vi "SyncedRecording.vi"() -> ()   [LabVIEW 2017]
doc: "I. Description:\nThis example demonstrates how to continuously acquire and generate data at the same time, synchronized with one another.\n\nII. Instructions for Running:\n1. Select the physical channel to correspond to where your signal is input on the DAQ device. Also, select the corresponding channel for where your signal is being generated.\n2. Enter the minimum and maximum voltage ranges.\nNote: For better accuracy try to match the input range to the expected voltage level of the measured signal.\n3. Set the sample rate of the acquisition.\nNote: The rate should be at least twice as fast as the maximum frequency component of the signal being acquired. \n6. Select the Rate for the generation\n7. Select what type of signal to generate and the amplitude.\nNote: This example requires two DMA channels to run. If your hardware does not support two DMA channels, you need to set the Data Transfer Mechanism property for the Analog Output Task to use \"Interrupts\". The Data Transfer Mechanism property is located in the DAQmx Channel Property hierarchy at:\n\nDAQmx Channel Property Node>>Analog Output>>General Properties>>Advanced>>Data Transfer and Memory>>Data Transfer Mechanism\n\nRefer to your device documentation to determine how many DMA channels are supported for your hardware.\n\nIII. Block Diagram Steps:\n1. Create an analog input voltage channel. Also, create an analog output voltage channel.\n2. Set the rate for the sample clock. Additionally, define the sample mode to be continuous. Also, set the sample clock rate for the signal generation.\n2a. Call the Get Terminal Name with Device Prefix VI. This will take a Task and a terminal and create a properly formatted device + terminal name to use as the source of the Trigger.\n3. Define the parameters for a Digital Edge Start Trigger. Set the Analog output to trigger off the AI Start Trigger. This is an internal trigger signal.\n4. Use the Basic Function Generator VI to create the signal to be generated.\n5. Call the Start VI to arm the two functions. Make sure the analog output is armed before the analog input. This will ensure both will start at the same time.\n6. Read the waveform data in a loop until the user hits the stop button or an error occurs. The Is Task Done? VI is used to check for errors in the Analog Output Task.\n7. Call the Clear VI to Clear the Task\n8. Use the popup dialog box to display an error if any.\n\nIV. I/O Connections Overview:\nMake sure your signal input/output terminals match the Physical Channel I/O controls."
uses:
  <vilib>/measure/NI_MABase.lvlib
panel:
  in  "Analog Input Sample Clock Source":tag="/Dev1/ao/SampleClock"
  out "Actual Update Generation Rate":dbl=5000.0 format="%0.2f"
  out "Actual Input Rate":dbl=10000.0 format="%0.2f"
  in  "Amplitude":dbl=1.0 format="%0.2p"
  in  "Signal Type":T1(ring)
  in  "rate":dbl=5000.0 caption="Update Generation Rate" format="%0.2f"
  in  "Samples to Read":i32=1000
  in  "minimum value":dbl=-10.0 caption="Output Minimum Value" format="%0.2f"
  in  "maximum value":dbl=10.0 caption="Output Maximum Value" format="%0.2f"
  in  "physical channels":tag="Dev1/ao0" caption="Output Physical Channels"
  in  "Maximum Value":dbl=10.0 caption="Input Maximum Value" format="%0.2f"
  in  "Minimum Value":dbl=-10.0 caption="Input Minimum Value" format="%0.2f"
  in  "Physical Channel":tag="Dev1/ai0" caption="Input Physical Channel"
  in  "Rate":dbl=10000.0 caption="Input Rate" format="%0.2f"
  out "Measurement":waveform(dbl)(graph)={"t0"=timestamp(3130175569.9063873 s since 1904-01-01), "dt"=9.999999999999999e-05, "Y"=[], "attributes"=variant("NI_ChannelName"=variant(string "Dev1/ai1"), "NI_UnitDescription"=variant(string "Volts"))}
  # "For instructions, select Help>>Show Context Help"
  # "Channel Parameters"
  # "Timing Parameters"
  # "Signal Generation"
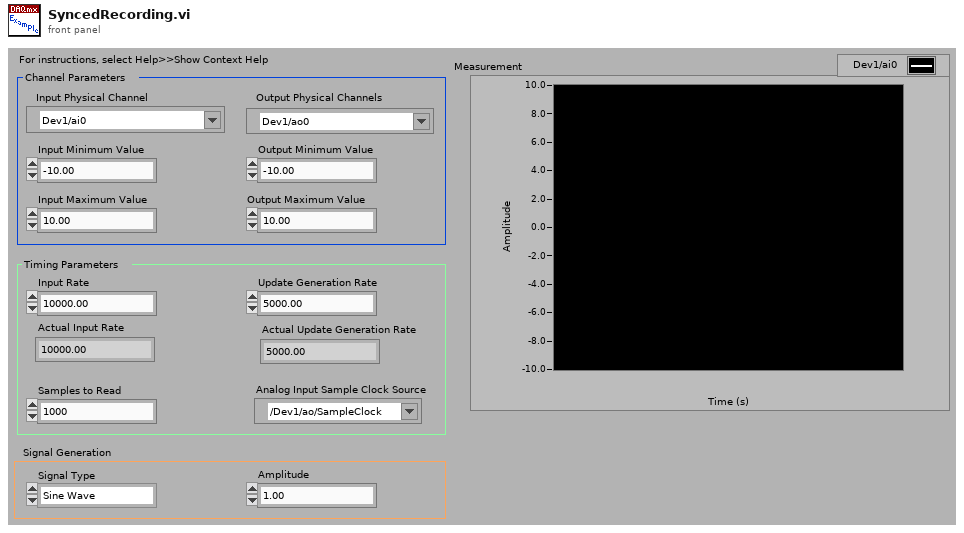
[diagram p1: front panel]
types:
  T1 = enum16{"Sine Wave", "Triangle Wave", "Square Wave", "Sawtooth Wave"}
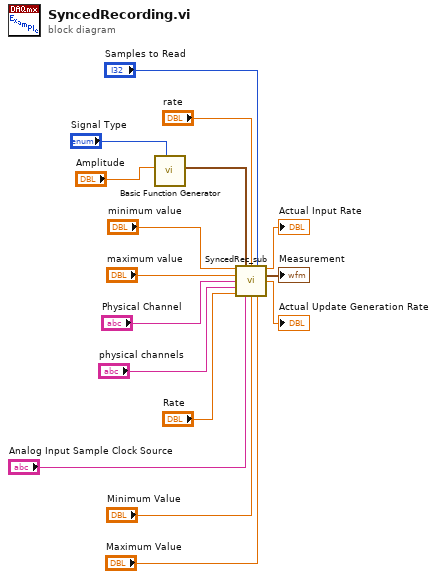
[diagram p0: block diagram]
diagram:
  n1 = call <vilib>:"Basic Function Generator.vi"("signal type"="Signal Type", "amplitude"="Amplitude") -> ("signal out"=w3:waveform(dbl))  [unwired: 7 in, 2 out]
  n2 = call "SyncedRec_sub.vi"("minimum value"="minimum value", "signal in"=w3, "rate"="rate", "Samples to Read"="Samples to Read", "maximum value"="maximum value", "Physical Channel"="Physical Channel", "physical channels"="physical channels", "Rate"="Rate", "Analog Input Sample Clock Source"="Analog Input Sample Clock Source", "Minimum Value"="Minimum Value", "Maximum Value"="Maximum Value") -> ("Actual Input Rate"=→"Actual Input Rate":dbl, "data"=→"Measurement":waveform(dbl), "Actual Update Generation Rate"=→"Actual Update Generation Rate":dbl)  [unwired: 2 in]
